vi "Assert Less_Variant.vi"(5 "Assert Only? (F)":bool, 6 "error code (1)":i32=1, 7 "Label":string, 8 "error in (no error)":errorcluster, 10 "Y":variant, 11 "X":variant) -> (0 "error out":errorcluster)   [LabVIEW 2009, in "Caraya.lvlib" / "Assert.lvclass"]
doc: "Generates an error if the input condition is not met.\n\n--\nCopyright © 2015 JKI All rights reserved.\n\nAuthor: Tomi Maila <tomi.maila@jki.net>\n\nThis library is provided \"AS IS\" ,WITHOUT WARRANTIES OR\nCONDITIONS OF ANY KIND, either express or implied.\n\nJKI -- jki.net"
uses:
  Assert.lvclass
panel:
  # "Copyright © 2015 JKI All rights reserved.\n\nAuthor: Tomi Maila <tomi.maila@jki.net>\n\nThis library is provided \"AS IS\" ,WITHOUT WARRANTIES OR\nCONDITIONS OF ANY KIND, either express or implied.\n\nJKI -- jki.net"
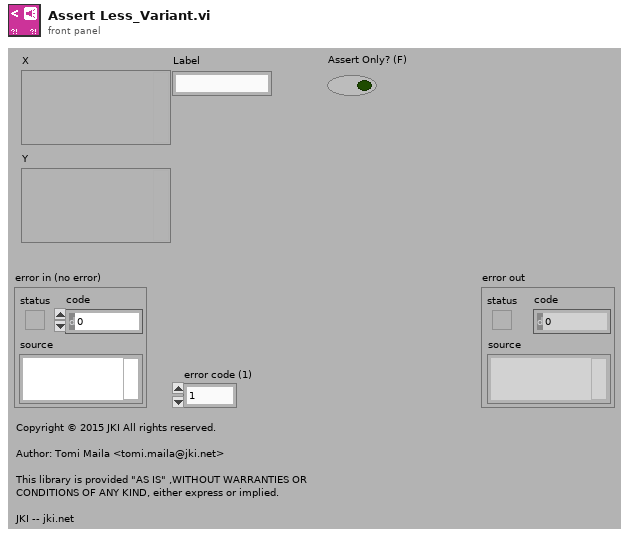
[diagram p1: front panel]
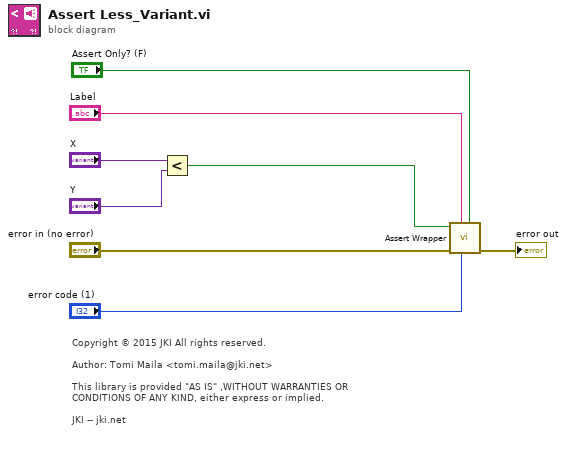
[diagram p0: block diagram]
diagram:
  # "Copyright © 2015 JKI All rights reserved.\n\nAuthor: Tomi Maila <tomi.maila@jki.net>\n\nThis library is provided \"AS IS\" ,WITHOUT WARRANTIES OR\nCONDITIONS OF ANY KIND, either express or implied.\n\nJKI -- jki.net"
  n1 = Less?(x="X", y="Y") -> (x < y?=w4:bool)
  n2 = call "Assert Wrapper.vi"("Assert Only? (F)"="Assert Only? (F)", "error code (1)"="error code (1)", "Label"="Label", "error in (no error)"="error in (no error)", "Assert?"=w4) -> ("error out"=→"error out":errorcluster)  [unwired: 6 in]
